vi "20220107_HW01.vi"() -> ()   [LabVIEW 2019]
uses:
  Status.ctl
panel:
  out "XY Graph":cluster{dbl[], dbl[]}[](graph)
  in  "Stop":bool
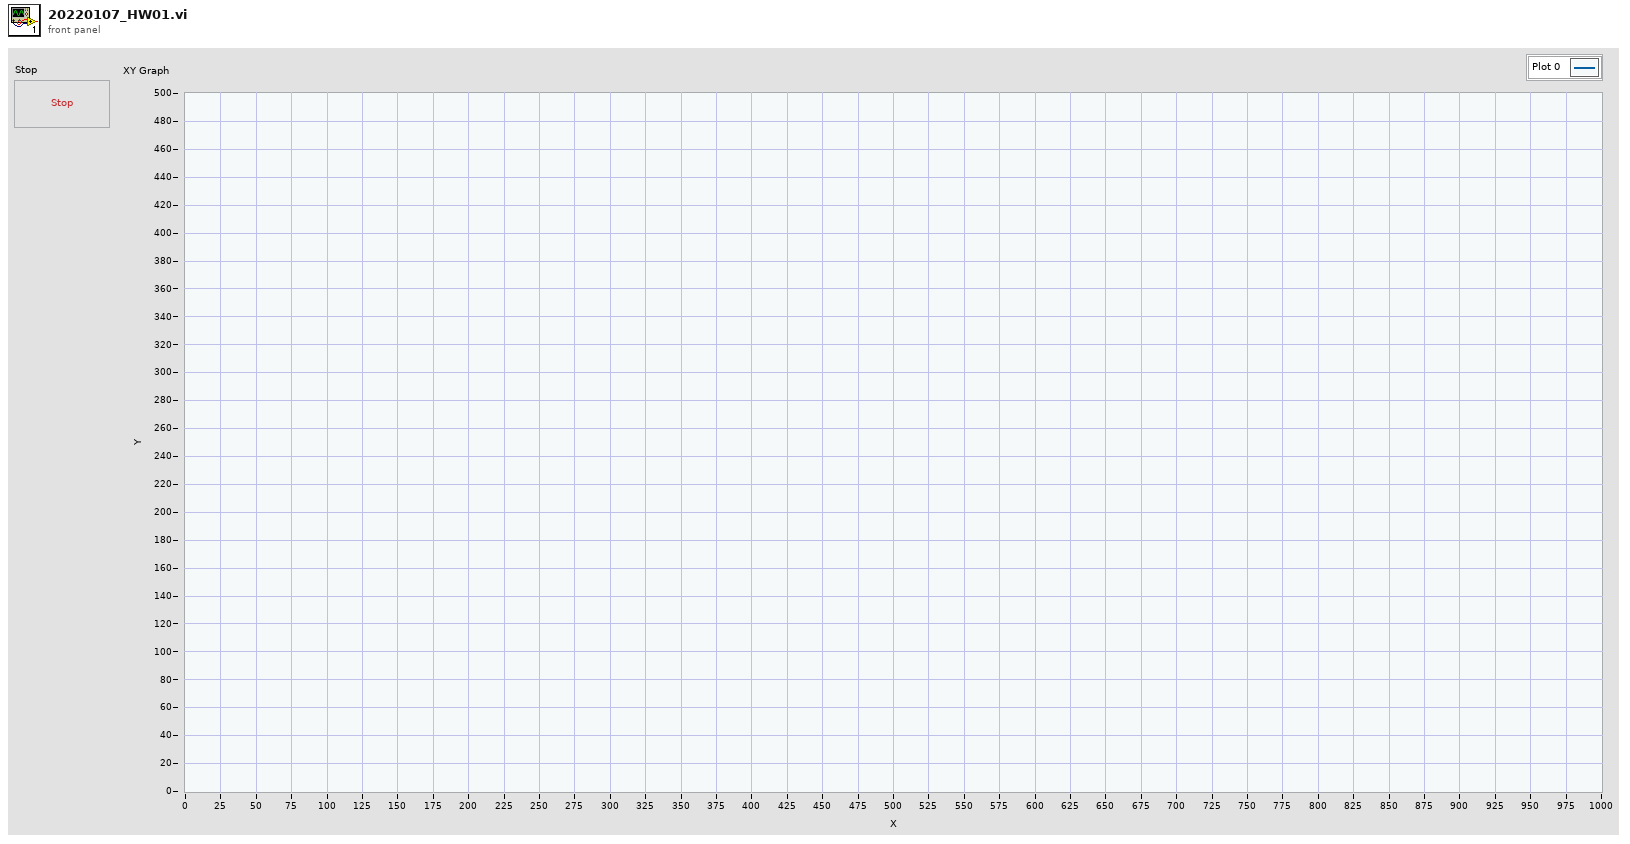
[diagram p1: front panel]
types:
  T1 = typedef "Status.ctl" = enum16{"Idle", "Add Point", "Move"}
  T2 = typedef "LVPoint32TypeDef.ctl" = cluster{"Horizontal":i32, "Vertical":i32}
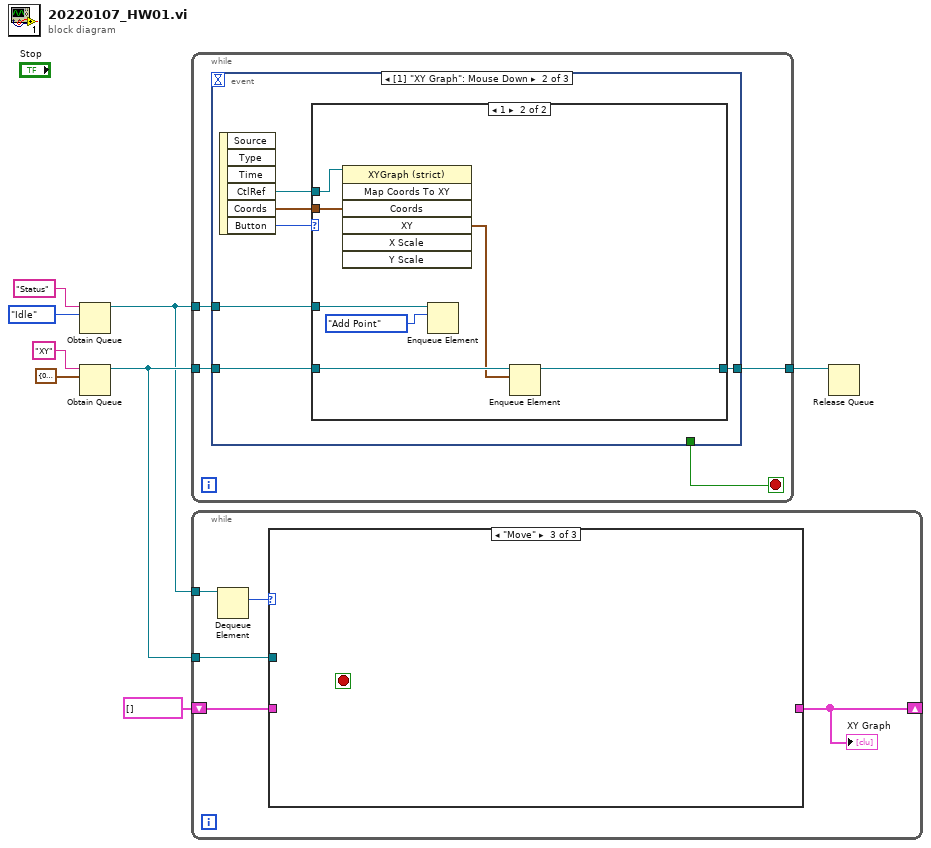
[diagram p0: block diagram]
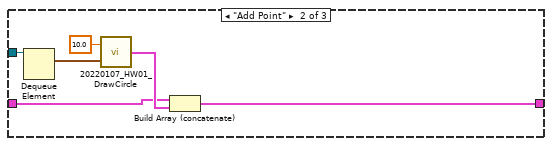
[diagram p3: hidden frame]
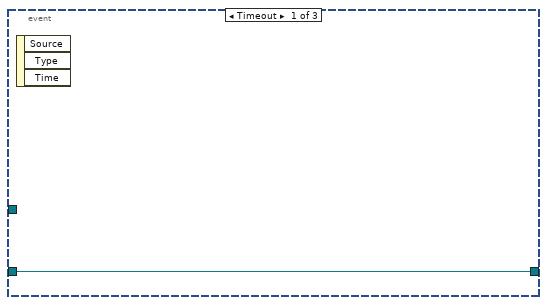
[diagram p4: hidden frame]
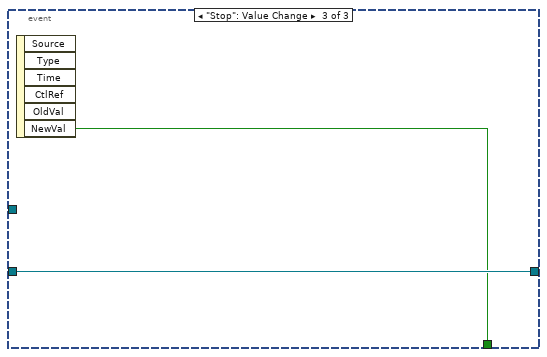
[diagram p6: hidden frame]
diagram:
  n1 = Obtain Queue(name (unnamed)="Status", element data type=Status."Idle") -> (queue out=w1:refnum<queue>)  [unwired: 3 in, 2 out]
  n2 = Obtain Queue(name (unnamed)="XY", element data type=cluster{"X":dbl, "Y":dbl} {"X"=0.0, "Y"=0.0} ("XY")) -> (queue out=w6:refnum<queue>)  [unwired: 3 in, 2 out]
  n3 = while {
    tunnel: w6 -> [w12]
    tunnel: [w10] -> w7
    tunnel: w1 -> [w9]
    stop <- w11 stop-if-true
    n4 = event shown="[1] \"XY Graph\": Mouse Down" {
      selector: _ -> [_ _ _]
      dyn-events: _ -> [_ _ _]
      timeout: _ -> [_ _ _]
      tunnel: w12 -> [w13 w18 w29]
      tunnel: [w13 w17 w29] -> w10
      tunnel: [_ _ w28] -> w11
      tunnel: w9 -> [_ w14 _]
      event Timeout {
        n5 = event-data() -> ()  [unwired: 1 in, 3 out]
      }
      event "XY Graph": Mouse Down {
        n6 = event-data() -> ("CtlRef"=w16:refnum<vi>, "Coords"=w15:T2, "Button"=w19:u16)  [unwired: 1 in, 3 out]
        n7 = case shown="1" w19 {
          tunnel: w18 -> [w20 w27]
          tunnel: [w20 w26] -> w17
          tunnel: w16 -> [_ w25]
          tunnel: w15 -> [_ w24]
          tunnel: w14 -> [_ w23]
          frame 0, Default {
          }
          frame 1 {
            n8 = invoke class="XYGraph (strict)" method="Map Coords To XY"(reference=w25, "Coords"=w24) -> ("XY"=w21:cluster{"X":dbl, "Y":dbl})  [unwired: 5 in, 6 out]
            n9 = Enqueue Element(queue=w23, element=Status."Add Point") -> ()  [unwired: 2 in, 3 out]
            n10 = Enqueue Element(queue=w27, element=w21) -> (queue out=w26:refnum<queue>)  [unwired: 2 in, 2 out]
          }
        }
      }
      event "Stop": Value Change {
        n11 = event-data() -> ("NewVal"=w28:bool)  [unwired: 1 in, 5 out]
      }
    }
  }
  n12 = while {
    tunnel: w6 -> [w34]
    shift-right: [w32] -> _
    shift-left: cluster{dbl[], dbl[]}[] [] -> [w33]
    tunnel: w1 -> [w31]
    stop <- _ stop-if-true
    n13 = Dequeue Element(queue=w31) -> (element=w30:T1)  [unwired: 2 in, 3 out]
    n14 = case shown="\"Move\"" w30 {
      tunnel: w34 -> [_ w41 _]
      tunnel: w33 -> [w35 w37 _]
      tunnel: [w35 w36 _] -> w32
      frame "Idle", Default {
      }
      frame "Add Point" {
        n15 = Dequeue Element(queue=w41) -> (element=w40:cluster{"X":dbl, "Y":dbl})  [unwired: 2 in, 3 out]
        n16 = call "20220107_HW01_DrawCircle.vi"("Offset"=w40, "Radius"=10.0) -> ("XY Graph"=w38:cluster{dbl[], dbl[]})
        n17 = Build Array (concatenate)(w37, w38) -> (w36:cluster{dbl[], dbl[]}[])
      }
      frame "Move" {
      }
    }
    "XY Graph" <- w32
  }
  n18 = Release Queue(queue=w7) -> ()  [unwired: 2 in, 3 out]
